vi "Keep true until....vi"(1 "Changer":bool, 2 "Keep":bool) -> (0 "Value":bool)   [LabVIEW 2012]
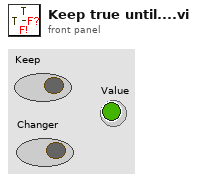
[diagram p1: front panel]
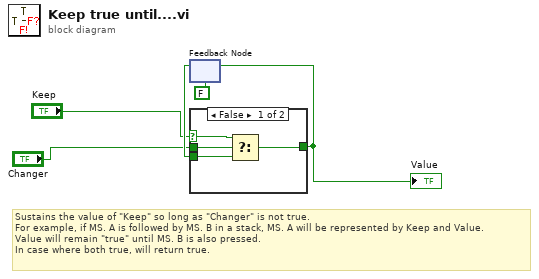
[diagram p0: block diagram]
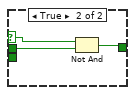
[diagram p2: hidden frame]
diagram:
  # "Sustains the value of \"Keep\" so long as \"Changer\" is not true.\nFor example, if MS. A is followed by MS. B in a stack, MS. A will be represented by Keep and Value.\nValue will remain \"true\" until MS. B is also pressed.\nIn case where both true, will return true."
  n1 = feedback #1(FALSE) -> (w4:bool)
  n2 = case shown="False" "Keep" {
    selector: "Keep" -> [w7 w12]
    tunnel: [w9 w11] -> w5
    tunnel: w4 -> [w8 _]
    tunnel: "Changer" -> [w6 w10]
    frame False {
      n3 = Select(t=w7, s=w6, f=w8) -> (s? t:f=w9:bool)
    }
    frame True {
      n4 = Not And(1:w10, 2:w12) -> (0:w11:bool)
    }
  }
  "Value" <- w5
  n5 = feedback-in #1(w5) -> ()
